vi "calibration file.vi"(0 "refnum in":refnum<k5>, 5 "Scaling":T2={"conversion matrix"=[[0.0, 0.0], [0.0, 0.0], [0.0, 0.0], [0.0, 0.0], [0.0, 0.0], [0.0, 0.0]], "units"="", "name"="", "scale type"=enum."Volts", "offset (volts)"=0.0, "second channel"=0, "correspondence table"=[], "offset (physical units)"=0.0, "pH scale"={"Buffers"=[], "Temperature"=0.0}, "D.O."={"Temperature"=0.0, "K"=0.0, "barometric pressure"=0.0}} {"D.O."."K" format="%.6f"; "D.O."."Temperature" format="%.2f"; "pH scale"."Buffers"."V/T" format="%.5f"; "pH scale"."Buffers"."Buffer" format="%.2f"; "pH scale"."Temperature" format="%.2f"; "offset (physical units)" format="%.5f"; "correspondence table"."volts" format="%.4f"; "correspondence table"."physical units" format="%.4f"; "second channel" min=-1; "offset (volts)" format="%.5f"; "conversion matrix" format="%.4e"}, 9 "method":T7={"sampling interval"=0.1, "samples to average"=1, "data interval"=0.0, "stream data"=FALSE, "file path"=refnum, "command"={"command"=enum."Idle", "start time (ms)"=0, "Channel Indices"=[], "Scans per Sample"=1}} {"command"."Scans per Sample" min=1; "data interval" format="%.2f"; "samples to average" min=1 step=1; "sampling interval" format="%.2f"}, 11 "Server Stats":T10={"scan rate"=10.0, "# connections"=0, "channel settings"=[]} {"channel settings"."lower input limits" format="%.4f"; "channel settings"."upper input limits" format="%.4f"; "scan rate" format="%.2f"}) -> (6 "Scaling out":T2={"conversion matrix"=[[0.0, 0.0], [0.0, 0.0], [0.0, 0.0], [0.0, 0.0], [0.0, 0.0], [0.0, 0.0]], "units"="", "name"="", "scale type"=enum."Volts", "offset (volts)"=0.0, "second channel"=0, "correspondence table"=[], "offset (physical units)"=0.0, "pH scale"={"Buffers"=[], "Temperature"=0.0}, "D.O."={"Temperature"=0.0, "K"=0.0, "barometric pressure"=0.0}} {"D.O."."K" format="%.6f"; "D.O."."Temperature" format="%.2f"; "pH scale"."Buffers"."V/T" format="%.5f"; "pH scale"."Buffers"."Buffer" format="%.2f"; "pH scale"."Temperature" format="%.2f"; "offset (physical units)" format="%.5f"; "correspondence table"."volts" format="%.4f"; "correspondence table"."physical units" format="%.4f"; "second channel" min=-1; "offset (volts)" format="%.5f"; "conversion matrix" format="%.4e"}, 15 "canceled":bool=TRUE)   [LabVIEW 2010]
uses:
  conversion.ctl
  DAQ configuration/scale type.ctl
  correspondence table.ctl
  DataServer/Server stats.ctl
  DataServer/command.ctl
  DataServer/command cluster.ctl
  DAC apps/support/method.ctl
  calib array.ctl
  pH/pH scale.ctl
  Dissolved Oxygen/DO scale.ctl
panel:
  in  "Calibration volts":T1=[{"conversion matrix"=[[0.0, 0.0], [0.0, 0.0], [0.0, 0.0], [0.0, 0.0], [0.0, 0.0], [0.0, 0.0]], "units"="", "name"="", "scale type"=enum."Volts", "offset (volts)"=0.0, "second channel"=0, "correspondence table"=[], "offset (physical units)"=0.0, "pH scale"={"Buffers"=[], "Temperature"=0.0}, "D.O."={"Temperature"=0.0, "K"=0.0, "barometric pressure"=0.0}}] {"D.O."."K" format="%.6f"; "D.O."."Temperature" format="%.2f"; "pH scale"."Buffers"."V/T" format="%.5f"; "pH scale"."Buffers"."Buffer" format="%.2f"; "pH scale"."Temperature" format="%.2f"; "offset (physical units)" format="%.5f"; "correspondence table"."volts" format="%.4f"; "correspondence table"."physical units" format="%.4f"; "second channel" min=-1; "offset (volts)" format="%.5f"; "conversion matrix" format="%.4e"}
  in  "cancel":bool
  in  "OK":bool
  in  "State":T11
  # "C"
  # "kPa"
  # "C"
  # "s"
  # "s"
  # "Hz"
  # "C"
  # "kPa"
  # "C"
  # "C"
  # "kPa"
  # "C"
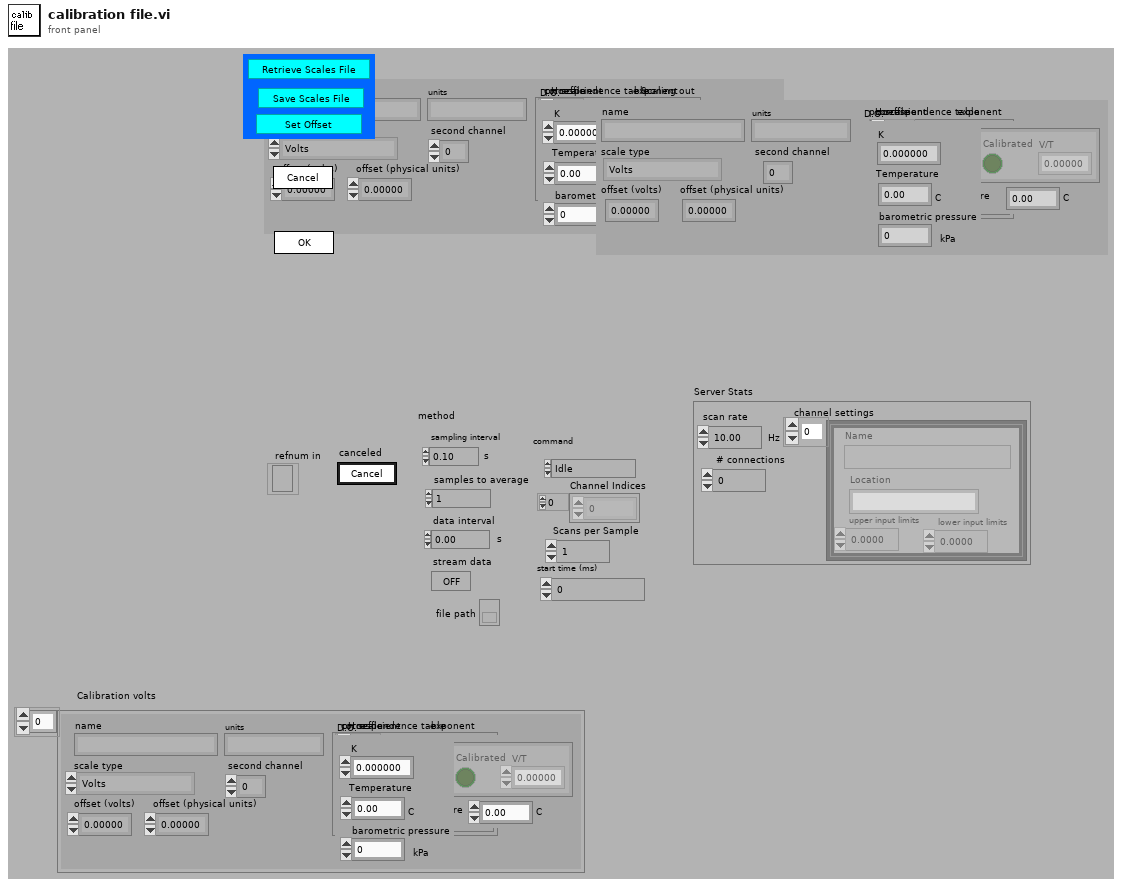
[diagram p1: front panel]
types:
  T1 = typedef "calib array.ctl" = T2[]
  T2 = typedef "conversion.ctl" = cluster{"conversion matrix":sgl[][], "units":string, "name":string, "scale type":T3, "offset (volts)":dbl, "second channel":i8, "correspondence table":T4, "offset (physical units)":dbl, "pH scale":T5, "D.O.":T6}
  T3 = typedef "scale type.ctl" = enum16{"Volts", "Polynomial", "Correspondence Table", "pH", "Dissolved Oxygen", "Quadratic"}
  T4 = typedef "correspondence table.ctl" = cluster{"physical units":dbl, "volts":dbl}[]
  T5 = typedef "pH scale.ctl" = cluster{"Buffers":cluster{"Buffer":dbl, "Calibrated":bool, "V/T":dbl}[], "Temperature":dbl}
  T6 = typedef "DO scale.ctl" = cluster{"Temperature":dbl, "K":dbl, "barometric pressure":dbl}
  T7 = typedef "method.ctl" = cluster{"sampling interval":sgl, "samples to average":u32, "data interval":sgl, "stream data":bool, "file path":refnum<file>, "command":T8}
  T8 = typedef "command cluster.ctl" = cluster{"command":T9, "start time (ms)":u32, "Channel Indices":i32[], "Scans per Sample":i32}
  T9 = typedef "command.ctl" = enum16{"Idle", "Send Data", "Send 1 Scan", "Logoff"}
  T10 = typedef "Server stats.ctl" = cluster{"scan rate":dbl, "# connections":i32, "channel settings":cluster{"Name":string, "upper input limits":sgl, "lower input limits":sgl, "Location":string}[]}
  T11 = cluster{"retrieve file":bool, "Save File":bool, "Set Offset":bool}
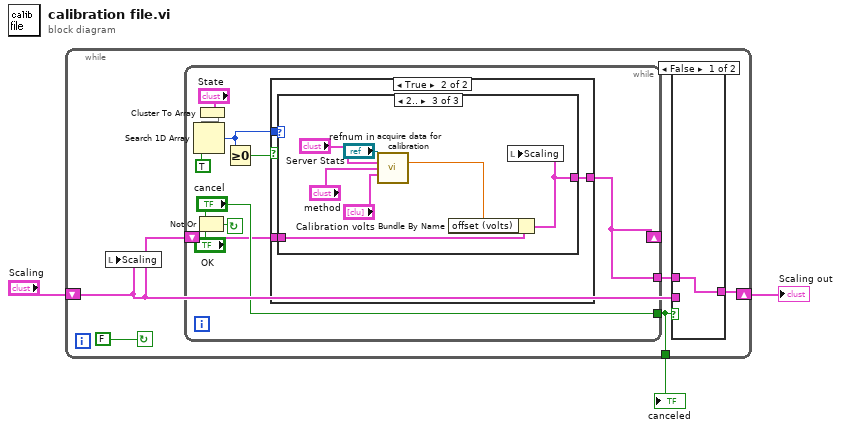
[diagram p0: block diagram]
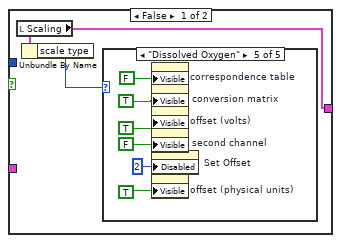
[diagram p2: hidden frame]
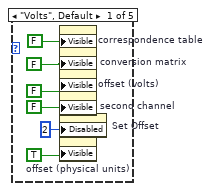
[diagram p3: hidden frame]
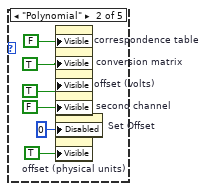
[diagram p4: hidden frame]
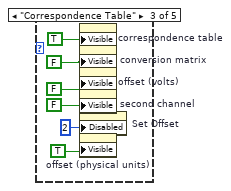
[diagram p5: hidden frame]
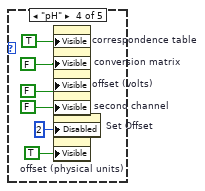
[diagram p6: hidden frame]
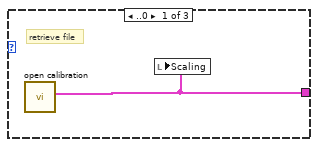
[diagram p7: hidden frame]
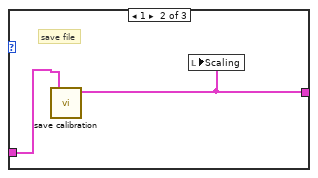
[diagram p8: hidden frame]
diagram:
  n1 = while {
    tunnel: [w6] -> w3
    shift-left: "Scaling" -> [w5]
    shift-right: [w8] -> w2
    stop <- FALSE continue-if-true
    n2 = local write "Scaling"(w5) -> ()
    n3 = while {
      shift-left: w5 -> [w10]
      shift-right: [w9] -> _
      tunnel: [w9] -> w7
      tunnel: ["cancel"] -> w6
      stop <- w13 continue-if-true
      n4 = Not Or(1:"OK", 2:"cancel") -> (0:w13:bool)
      n5 = Cluster To Array(cluster="State") -> (array=w14:bool[])
      n6 = Search 1D Array(1D array=w14, element=TRUE) -> (index of element=w17:i32)  [unwired: 1 in]
      n7 = Greater Or Equal To 0?(x=w17) -> (x >= 0?=w18:bool)
      n8 = case shown="True" w18 {
        tunnel: w17 -> [_ w53]
        tunnel: [w20 w52] -> w9
        tunnel: w10 -> [_ w51]
        frame False {
          n9 = local read "Scaling"() -> (w20:T2)
          n10 = Unbundle By Name(w20) -> ("scale type"=w19:T3)
          n11 = case shown="\"Dissolved Oxygen\"" w19 {
            frame "Volts", Default {
              n12 = property on="correspondence table" class="Arr (strict)"("Visible"=FALSE ("Write Attribute")) -> ()  [unwired: 2 in, 2 out]
              n13 = property on="conversion matrix" class="Arr (strict)"("Visible"=FALSE ("Write Attribute")) -> ()  [unwired: 2 in, 2 out]
              n14 = property on="offset (volts)" class="DigNum (strict)"("Visible"=FALSE ("Write Attribute")) -> ()  [unwired: 2 in, 2 out]
              n15 = property on="second channel" class="DigNum (strict)"("Visible"=FALSE ("Write Attribute")) -> ()  [unwired: 2 in, 2 out]
              n16 = property on="Set Offset" class="Bool"("Disabled"=u8 2 ("Write Attribute")) -> ()  [unwired: 2 in, 2 out]
              n17 = property on="offset (physical units)" class="DigNum (strict)"("Visible"=TRUE ("Write Attribute")) -> ()  [unwired: 2 in, 2 out]
            }
            frame "Polynomial" {
              n18 = property on="correspondence table" class="Arr (strict)"("Visible"=FALSE ("Write Attribute")) -> ()  [unwired: 2 in, 2 out]
              n19 = property on="conversion matrix" class="Arr (strict)"("Visible"=TRUE ("Write Attribute")) -> ()  [unwired: 2 in, 2 out]
              n20 = property on="offset (volts)" class="DigNum (strict)"("Visible"=TRUE ("Write Attribute")) -> ()  [unwired: 2 in, 2 out]
              n21 = property on="second channel" class="DigNum (strict)"("Visible"=FALSE ("Write Attribute")) -> ()  [unwired: 2 in, 2 out]
              n22 = property on="Set Offset" class="Bool"("Disabled"=u8 0 ("Write Attribute")) -> ()  [unwired: 2 in, 2 out]
              n23 = property on="offset (physical units)" class="DigNum (strict)"("Visible"=TRUE ("Write Attribute")) -> ()  [unwired: 2 in, 2 out]
            }
            frame "Correspondence Table" {
              n24 = property on="correspondence table" class="Arr (strict)"("Visible"=TRUE ("Write Attribute")) -> ()  [unwired: 2 in, 2 out]
              n25 = property on="conversion matrix" class="Arr (strict)"("Visible"=FALSE ("Write Attribute")) -> ()  [unwired: 2 in, 2 out]
              n26 = property on="offset (volts)" class="DigNum (strict)"("Visible"=FALSE ("Write Attribute")) -> ()  [unwired: 2 in, 2 out]
              n27 = property on="second channel" class="DigNum (strict)"("Visible"=FALSE ("Write Attribute")) -> ()  [unwired: 2 in, 2 out]
              n28 = property on="Set Offset" class="Bool"("Disabled"=u8 2 ("Write Attribute")) -> ()  [unwired: 2 in, 2 out]
              n29 = property on="offset (physical units)" class="DigNum (strict)"("Visible"=TRUE ("Write Attribute")) -> ()  [unwired: 2 in, 2 out]
            }
            frame "pH" {
              n30 = property on="correspondence table" class="Arr (strict)"("Visible"=TRUE ("Write Attribute")) -> ()  [unwired: 2 in, 2 out]
              n31 = property on="conversion matrix" class="Arr (strict)"("Visible"=FALSE ("Write Attribute")) -> ()  [unwired: 2 in, 2 out]
              n32 = property on="offset (volts)" class="DigNum (strict)"("Visible"=FALSE ("Write Attribute")) -> ()  [unwired: 2 in, 2 out]
              n33 = property on="second channel" class="DigNum (strict)"("Visible"=FALSE ("Write Attribute")) -> ()  [unwired: 2 in, 2 out]
              n34 = property on="Set Offset" class="Bool"("Disabled"=u8 2 ("Write Attribute")) -> ()  [unwired: 2 in, 2 out]
              n35 = property on="offset (physical units)" class="DigNum (strict)"("Visible"=TRUE ("Write Attribute")) -> ()  [unwired: 2 in, 2 out]
            }
            frame "Dissolved Oxygen" {
              n36 = property on="correspondence table" class="Arr (strict)"("Visible"=FALSE ("Write Attribute")) -> ()  [unwired: 2 in, 2 out]
              n37 = property on="conversion matrix" class="Arr (strict)"("Visible"=TRUE ("Write Attribute")) -> ()  [unwired: 2 in, 2 out]
              n38 = property on="offset (volts)" class="DigNum (strict)"("Visible"=TRUE ("Write Attribute")) -> ()  [unwired: 2 in, 2 out]
              n39 = property on="second channel" class="DigNum (strict)"("Visible"=FALSE ("Write Attribute")) -> ()  [unwired: 2 in, 2 out]
              n40 = property on="Set Offset" class="Bool"("Disabled"=u8 2 ("Write Attribute")) -> ()  [unwired: 2 in, 2 out]
              n41 = property on="offset (physical units)" class="DigNum (strict)"("Visible"=TRUE ("Write Attribute")) -> ()  [unwired: 2 in, 2 out]
            }
          }
        }
        frame True {
          n42 = Greater Or Equal To 0?(x=w53) -> ()  [unwired: 1 out]
          n43 = case shown="2.." w53 {
            tunnel: [w54 w55 w57] -> w52
            tunnel: w51 -> [_ w56 w60]
            frame ..0 {
              # "retrieve file"
              n44 = call "open calibration.vi"() -> ("conversion out"=w54:T2)  [unwired: 7 in]
              n45 = local write "Scaling"(w54) -> ()
            }
            frame 1 {
              # "save file"
              n46 = call "save calibration.vi"("conversion in"=w56) -> ("conversion out"=w55:T2)  [unwired: 6 in]
              n47 = local write "Scaling"(w55) -> ()
            }
            frame 2.. {
              n48 = call "acquire data for calibration.vi"("Connection ID"="refnum in", 5:"Server Stats", "method"="method", "Reference Index"="Calibration volts") -> ("offset"=w59:sgl)  [unwired: 9 in, 2 out]
              n49 = Bundle By Name(cluster=w60, "offset (volts)"=w59) -> (w57:T2)
              n50 = local write "Scaling"(w57) -> ()
            }
          }
        }
      }
    }
    n51 = case shown="False" w6 {
      tunnel: w5 -> [_ w65]
      tunnel: [w64 w65] -> w8
      tunnel: w7 -> [w64 _]
      frame False {
      }
      frame True {
      }
    }
  }
  "canceled" <- w3
  "Scaling out" <- w2
